vi "GUI_Preamp2_delay.vi"(8 "error IO":errorcluster) -> (0 "error IO 2":errorcluster)   [LabVIEW 2013]
uses:
  shared programs/GUI_Template/GUI_master/tcp_new_data_event.ctl
  shared programs/GUI_Template/GUI_master/tcp new data cluster.ctl
  DelayControl_For Multiple Channels.ctl
  channels_TypDef.ctl
  General/Device GUIs/GUI_DG645/DelayControl2.ctl
  VIremote/VIremote.llb/VIremoteFunction.ctl
panel:
  in  "insert tag":bool=TRUE
  in  "stop":bool
  out "status":bool
  in  "reference.Channel_D::2":string caption="reference.Channel_A::2"
  in  "reference.Channel_C::2":string caption="reference.Channel_A::2"
  in  "reference.Channel_B::2":string caption="reference.Channel_A::2"
  in  "delay.Channel_D::2":dbl=0.001 caption="Q Switch Delay" min=0.0 max=1.0 format="%_12f"
  in  "delay.Channel_C::2":dbl=0.001 caption="Q Switch Delay" min=0.0 max=1.0 format="%_12f"
  in  "Delay.Ch D":T1={"Channel"="D", "Linked"=enum."T0", "Delay"=0.0} {"Delay" format="%+.12f"}
  in  "Delay.Ch C":T1={"Channel"="C", "Linked"=enum."T0", "Delay"=0.0} {"Delay" format="%+.12f"}
  in  "Delay.Ch B":T1={"Channel"="B", "Linked"=enum."T0", "Delay"=0.0} {"Delay" format="%+.12f"}
  in  "reference.Channel_A::2":string
  in  "Delay.Ch A":T1={"Channel"="A", "Linked"=enum."T0", "Delay"=0.0} {"Delay" format="%+.12f"}
  in  "delay.Channel_A::2":dbl=0.001 caption="Lamp Delay" min=0.0 max=1.0 format="%_12f"
  in  "delay.Channel_B::2":dbl=0.001 caption="Q Switch Delay" min=0.0 max=1.0 format="%_12f"
  in  "GUIdevice 2":string="TREX-Preamp2Delay"
  out "tcp data event":T4
  # "Preamp 2"
  # "in meters..."
  # "="
  # "="
  # "="
  # "="
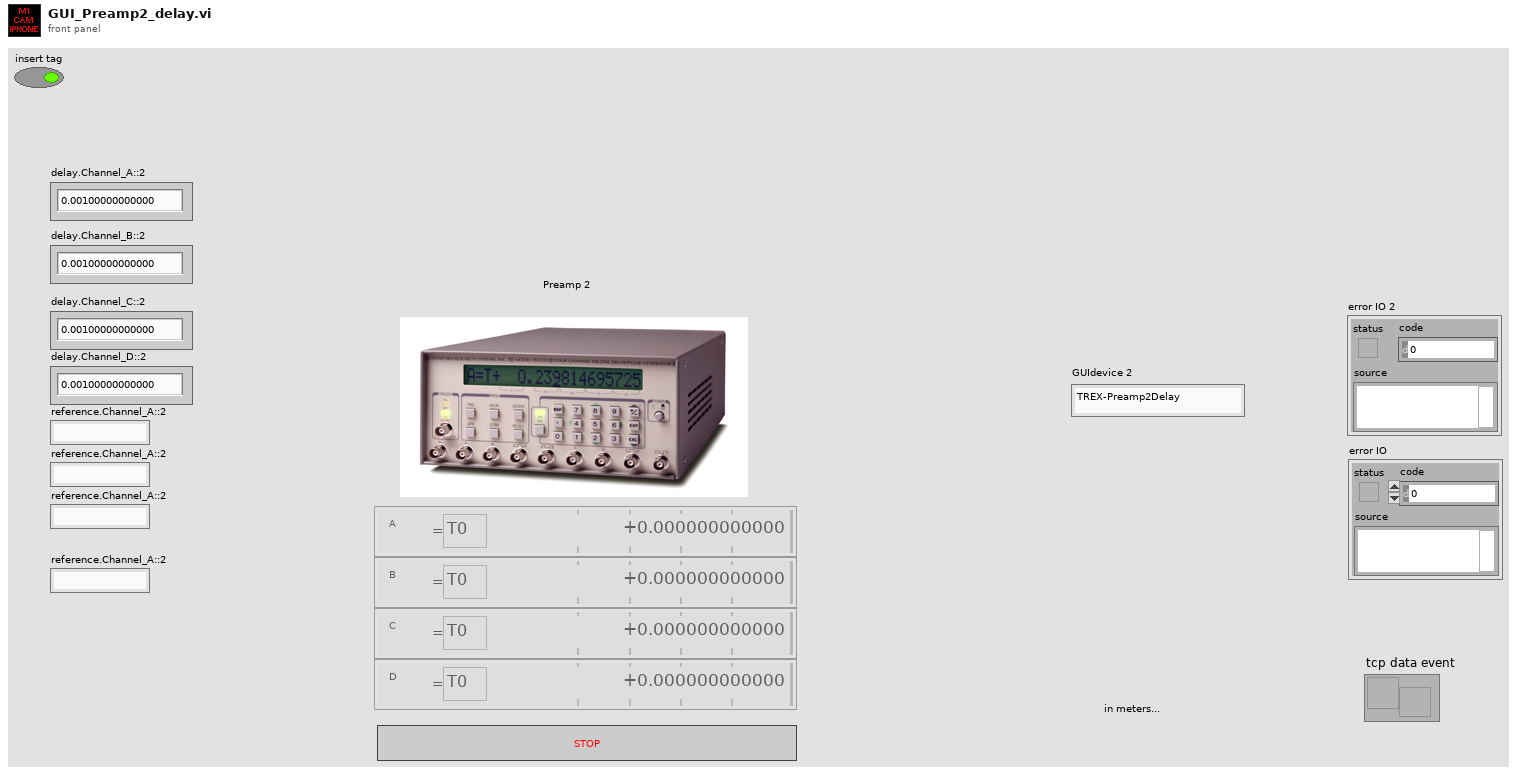
[diagram p1: front panel]
types:
  T1 = typedef "DelayControl_For Multiple Channels.ctl" = cluster{"Channel":string, "Linked":T2, "Delay":T3}
  T2 = typedef "channels_TypDef.ctl" = enum16{"T0", "A", "B", "C", "D"}
  T3 = typedef "DelayControl2.ctl" = dbl
  T4 = typedef "tcp_new_data_event.ctl" = refnum<user-event>
  T5 = typedef "tcp new data cluster.ctl" = cluster{"EventEnum":enum16{"new data", "connection status update"}, "Device name":string}
  T6 = typedef "VIremoteFunction.ctl" = enum16{"Do nothing", "Stop controller", "Close this connection", "Show info panel", "Set VI to control", "Set Accelerometer freq (Hz)", "Show Alert message", "Start Sound Input", "Stop Sound Input", "Set Volume (0-100)", "Set sound output Speaker", "Set sound output Receiver", "Play Sound", "Repeat Sound", "Stop Sound", "Pause Sound", "Resume Sound", "Set panel width of caller (320 or 480)", "Set Panel Size to Portrait", "Set Panel Size to Landscape", "Set Panel Size as Current Orientation", "Allow all UI Orientations", "Send user notification", "Disable Scrolling", "Normal Scrolling", "Page Scrolling", "Set Scroll Offset", "Page Indicator Position"}
  T7 = enum8{"Enabled", "Disabled", "Disabled and Grayed Out"}
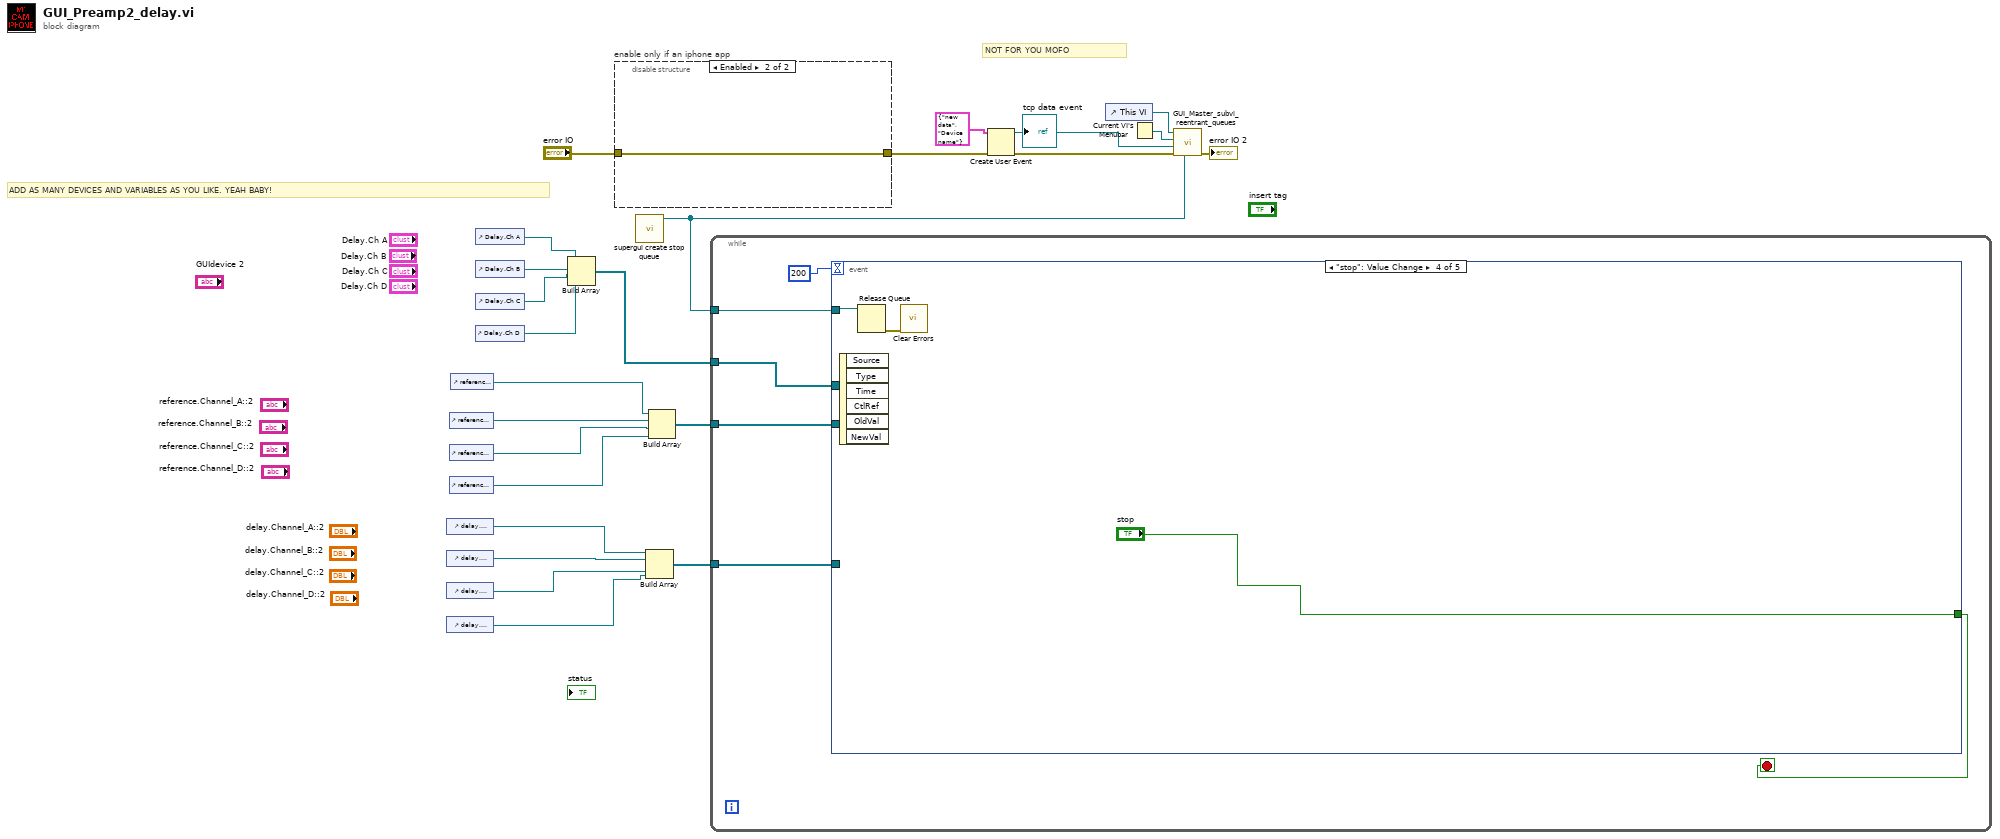
[diagram p0: block diagram]
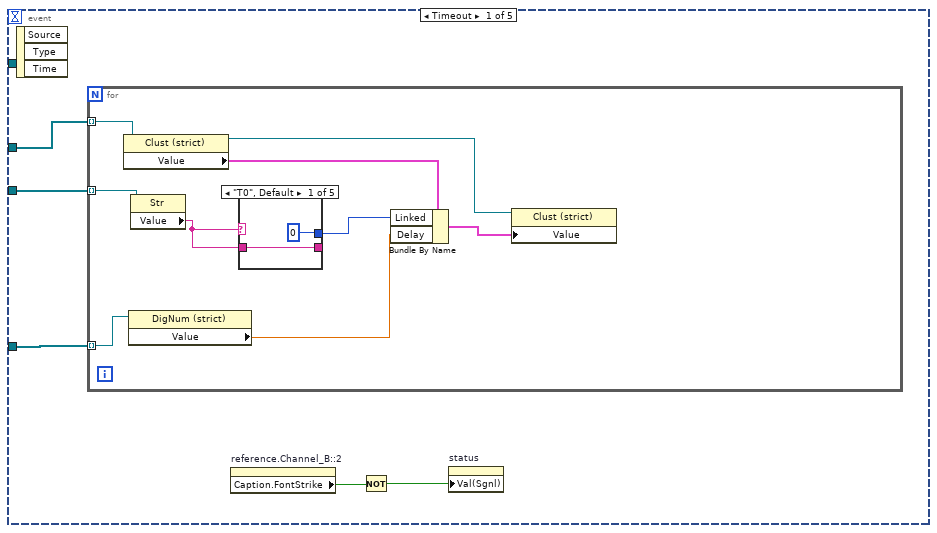
[diagram p2: hidden frame]
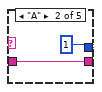
[diagram p3: hidden frame]
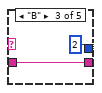
[diagram p4: hidden frame]
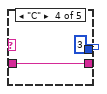
[diagram p5: hidden frame]
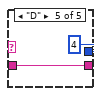
[diagram p6: hidden frame]
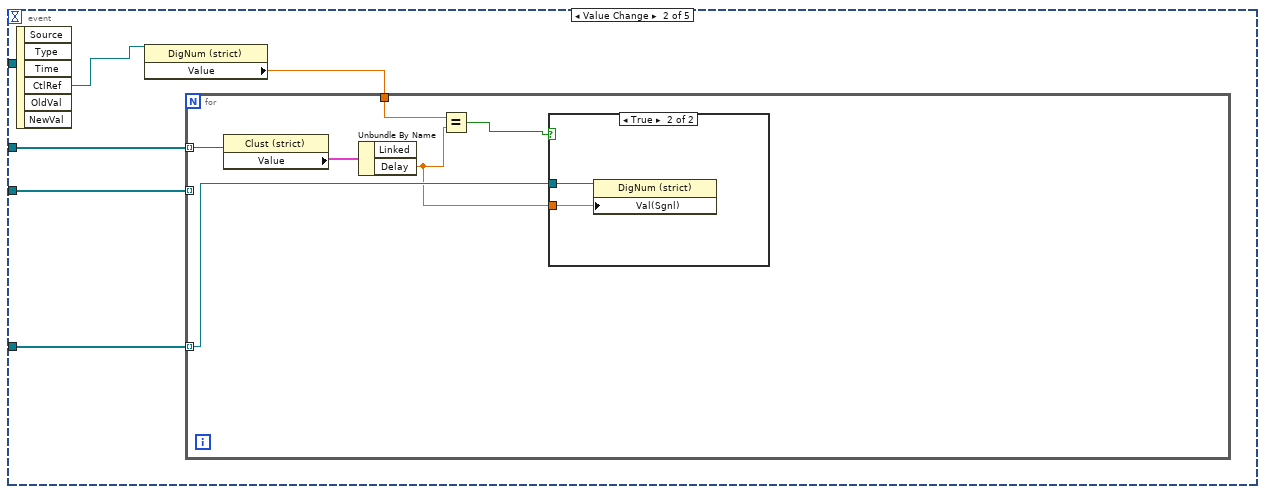
[diagram p7: hidden frame]
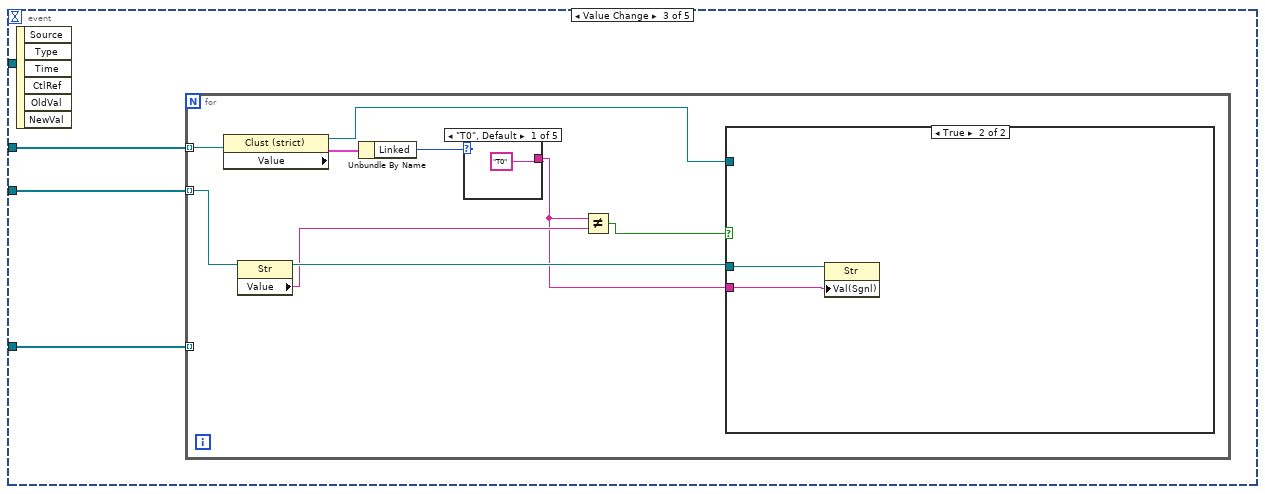
[diagram p9: hidden frame]
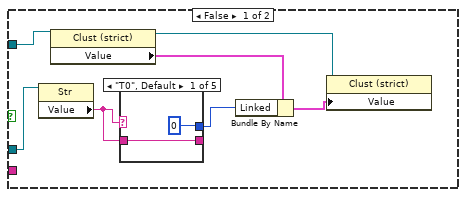
[diagram p10: hidden frame]
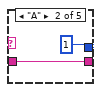
[diagram p11: hidden frame]
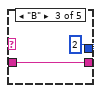
[diagram p12: hidden frame]
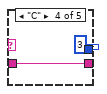
[diagram p13: hidden frame]
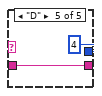
[diagram p14: hidden frame]
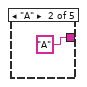
[diagram p15: hidden frame]
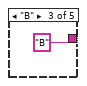
[diagram p16: hidden frame]
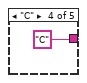
[diagram p17: hidden frame]
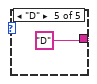
[diagram p18: hidden frame]
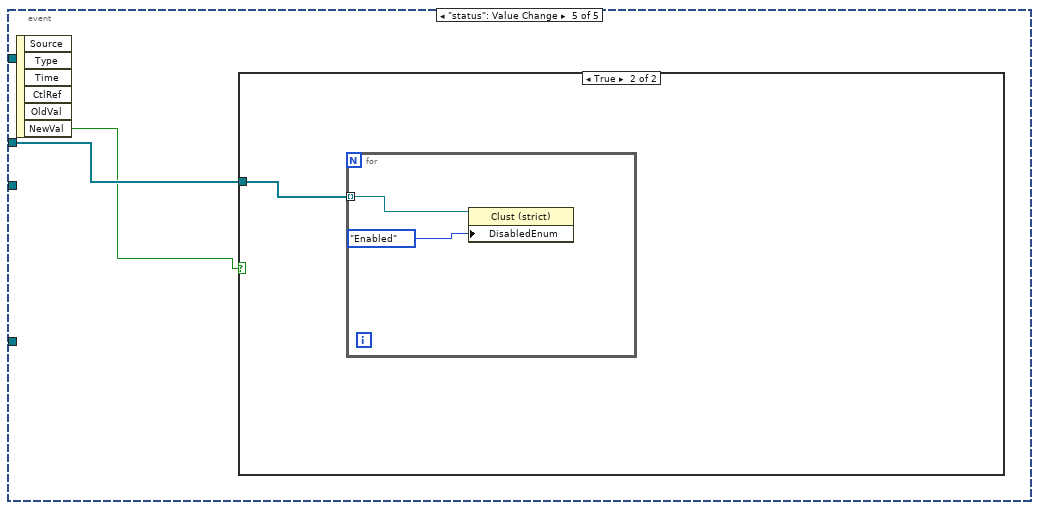
[diagram p19: hidden frame]
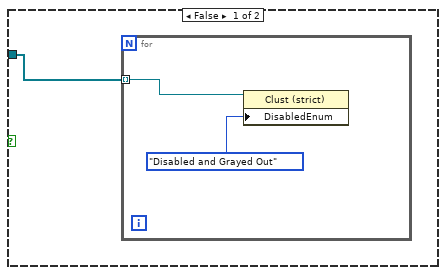
[diagram p20: hidden frame]
diagram:
  # "NOT FOR YOU MOFO"
  # "ADD AS MANY DEVICES AND VARIABLES AS YOU LIKE. YEAH BABY!"
  n1 = control-ref of="delay.Channel_A::2"() -> (w13:refnum<vi>)
  n2 = control-ref of="delay.Channel_B::2"() -> (w12:refnum<vi>)
  n3 = control-ref of="delay.Channel_C::2"() -> (w11:refnum<vi>)
  n4 = control-ref of="delay.Channel_D::2"() -> (w10:refnum<vi>)
  n5 = control-ref of="reference.Channel_B::2"() -> (w16:refnum<vi>)
  n6 = control-ref of="reference.Channel_C::2"() -> (w15:refnum<vi>)
  n7 = control-ref of="reference.Channel_D::2"() -> (w14:refnum<vi>)
  n8 = control-ref of="reference.Channel_A::2"() -> (w2:refnum<vi>)
  n9 = control-ref of="Delay.Ch A"() -> (w7:refnum<vi>)
  n10 = control-ref of="Delay.Ch B"() -> (w6:refnum<vi>)
  n11 = control-ref of="Delay.Ch C"() -> (w5:refnum<vi>)
  n12 = control-ref of="Delay.Ch D"() -> (w4:refnum<vi>)
  n13 = Build Array(w7, w6, w5, w4) -> (w3:refnum<vi>[])
  n14 = disable-structure "enable only if an iphone app" shown="Enabled" {
    disable-tunnel: [w26 w30] -> w19
    disable-tunnel: "error IO" -> [w25 w30]
    frame Disabled {
      n15 = call "VIremoteFunctions.vi"("error in (no error)"=w25, "Function"=VIremoteFunction."Set VI to control") -> ("error out"=w27:errorcluster)  [unwired: 4 in, 5 out]
      n16 = call "VIremoteFunctions.vi"("error in (no error)"=w27, "Function"=VIremoteFunction."Set Panel Size to Landscape") -> ("error out"=w26:errorcluster)  [unwired: 4 in, 5 out]
    }
    frame Enabled {
    }
  }
  n17 = call "supergui create stop queue.vi"() -> ("STOP Queue out"=w1:refnum<queue>)  [unwired: 11 in]
  n18 = Build Array(w13, w12, w11, w10) -> (w8:refnum<vi>[])
  n19 = Build Array(w2, w16, w15, w14) -> (w9:refnum<vi>[])
  n20 = while {
    tunnel: w9 -> [w34]
    tunnel: w8 -> [w33]
    tunnel: w3 -> [w32]
    tunnel: w1 -> [w31]
    stop <- w36 stop-if-true
    n21 = event shown="[3] \"stop\": Value Change" {
      selector: _ -> [_ _ _ _ _]
      dyn-events: _ -> [_ _ _ _ _]
      timeout: 200 -> [_ _ _ _ _]
      tunnel: [_ _ _ "stop" _] -> w36
      tunnel: w34 -> [w41 w64 w75 _ _]
      tunnel: w33 -> [w39 w63 w74 _ _]
      tunnel: w32 -> [w40 w65 w76 _ w114]
      tunnel: w31 -> [_ _ _ w111 _]
      event Timeout {
        n22 = event-data() -> ()  [unwired: 1 in, 3 out]
        n23 = for {
          tunnel: w41 -> [w50] mode=indexing
          tunnel: w40 -> [w49] mode=indexing
          tunnel: w39 -> [w45] mode=indexing
          n24 = property class="Clust (strict)"(reference=w49) -> (reference out=w42:refnum<vi>, "Value"=w47:T1)  [unwired: 1 in, 1 out]
          n25 = property class="DigNum (strict)"(reference=w45) -> ("Value"=w44:dbl)  [unwired: 1 in, 2 out]
          n26 = property class="Str"(reference=w50) -> ("Value"=w48:string)  [unwired: 1 in, 2 out]
          n27 = case shown="\"T0\", Default" w48 {
            tunnel: [0 1 2 3 4] -> w46
            tunnel: w48 -> [w51 w53 w55 w57 w59]
            tunnel: [w51 w53 w55 w57 w59] -> _
            frame "T0", Default {
            }
            frame "A" {
            }
            frame "B" {
            }
            frame "C" {
            }
            frame "D" {
            }
          }
          n28 = Bundle By Name(cluster=w47, "Linked"=w46, "Delay"=w44) -> (w43:T1)
          n29 = property class="Clust (strict)"(reference=w42, "Value"=w43) -> ()  [unwired: 1 in, 2 out]
        }
        n30 = property on="reference.Channel_B::2" class="Str"() -> ("Caption.FontStrike"=w38:bool)  [unwired: 2 in, 2 out]
        n31 = Not(x=w38) -> (.not. x?=w37:bool)
        n32 = property on="status" class="Bool (strict)"("Val(Sgnl)"=w37) -> ()  [unwired: 2 in, 2 out]
      }
      event Value Change {
        n33 = event-data() -> ("CtlRef"=w62:refnum<vi>)  [unwired: 1 in, 5 out]
        n34 = property class="DigNum (strict)"(reference=w62) -> ("Value"=w61:T3)  [unwired: 1 in, 2 out]
        n35 = for {
          tunnel: w65 -> [w69] mode=indexing
          tunnel: w64 -> [_] mode=indexing
          tunnel: w63 -> [w71] mode=indexing
          tunnel: w61 -> [w68]
          n36 = property class="Clust (strict)"(reference=w69) -> ("Value"=w70:T1)  [unwired: 1 in, 2 out]
          n37 = Unbundle By Name(w70) -> ("Delay"=w67:T3)  [unwired: 1 out]
          n38 = Equal?(x=w68, y=w67) -> (x = y?=w66:bool)
          n39 = case shown="True" w66 {
            tunnel: w71 -> [_ w73]
            tunnel: w67 -> [_ w72]
            frame False {
            }
            frame True {
              n40 = property class="DigNum (strict)"(reference=w73, "Val(Sgnl)"=w72) -> ()  [unwired: 1 in, 2 out]
            }
          }
        }
      }
      event Value Change {
        n41 = event-data() -> ()  [unwired: 1 in, 6 out]
        n42 = for {
          tunnel: w76 -> [w78] mode=indexing
          tunnel: w75 -> [w84] mode=indexing
          tunnel: w74 -> [_] mode=indexing
          n43 = property class="Clust (strict)"(reference=w78) -> (reference out=w77:refnum<vi>, "Value"=w79:T1)  [unwired: 1 in, 1 out]
          n44 = property class="Str"(reference=w84) -> (reference out=w83:refnum<vi>, "Value"=w82:string)  [unwired: 1 in, 1 out]
          n45 = Unbundle By Name(w79) -> ("Linked"=w85:T2)
          n46 = case shown="\"T0\", Default" w85 {
            tunnel: ["T0" "A" "B" "C" "D"] -> w80
            frame "T0", Default {
            }
            frame "A" {
            }
            frame "B" {
            }
            frame "C" {
            }
            frame "D" {
            }
          }
          n47 = Not Equal?(x=w80, y=w82) -> (x != y?=w81:bool)
          n48 = case shown="True" w81 {
            tunnel: w83 -> [w92 w104]
            tunnel: w80 -> [_ w103]
            tunnel: w77 -> [w86 _]
            frame False {
              n49 = property class="Str"(reference=w92) -> ("Value"=w90:string)  [unwired: 1 in, 2 out]
              n50 = property class="Clust (strict)"(reference=w86) -> (reference out=w88:refnum<vi>, "Value"=w91:T1)  [unwired: 1 in, 1 out]
              n51 = case shown="\"T0\", Default" w90 {
                tunnel: [0 1 2 3 4] -> w89
                tunnel: w90 -> [w93 w95 w97 w99 w101]
                tunnel: [w93 w95 w97 w99 w101] -> _
                frame "T0", Default {
                }
                frame "A" {
                }
                frame "B" {
                }
                frame "C" {
                }
                frame "D" {
                }
              }
              n52 = Bundle By Name(cluster=w91, "Linked"=w89) -> (w87:T1)
              n53 = property class="Clust (strict)"(reference=w88, "Value"=w87) -> ()  [unwired: 1 in, 2 out]
            }
            frame True {
              n54 = property class="Str"(reference=w104, "Val(Sgnl)"=w103) -> ()  [unwired: 1 in, 2 out]
            }
          }
        }
      }
      event "stop": Value Change {
        n55 = event-data() -> ()  [unwired: 1 in, 6 out]
        n56 = Release Queue(queue=w111) -> (error out=w110:errorcluster)  [unwired: 2 in, 2 out]
        n57 = call <vilib>:"Clear Errors.vi"("error in (no error)"=w110) -> ()  [unwired: 6 in, 1 out]
      }
      event "status": Value Change {
        n58 = event-data() -> ("NewVal"=w113:bool)  [unwired: 1 in, 5 out]
        n59 = case shown="True" w113 {
          tunnel: w114 -> [w115 w118]
          frame False {
            n60 = for {
              tunnel: w115 -> [w117] mode=indexing
              n61 = property class="Clust (strict)"(reference=w117, "DisabledEnum"=T7."Disabled and Grayed Out" ("Disabled")) -> ()  [unwired: 1 in, 2 out]
            }
          }
          frame True {
            n62 = for {
              tunnel: w118 -> [w120] mode=indexing
              n63 = property class="Clust (strict)"(reference=w120, "DisabledEnum"=T7."Enabled" ("Disabled")) -> ()  [unwired: 1 in, 2 out]
            }
          }
        }
      }
    }
  }
  n64 = Create User Event(user event datatype=T5 {"EventEnum"=enum."new data", "Device name"="Device name"} ("New Event"), error in=w19) -> (user event=w17:refnum<user-event>, error out=w20:errorcluster)
  "tcp data event" <- w17
  n65 = control-ref of="This VI"() -> (w23:refnum<vi>)
  n66 = Current VI's Menubar() -> (w22:refnum<k9>)
  n67 = call "GUI_Master_subvi_reentrant_queues.vi"("STOP Queue in"=w1, "error in (no error)"=w20, "tcp data event"=w17, "Caller menu reference"=w22, "Caller VI ref"=w23) -> ("error out"=→"error IO 2":errorcluster)  [unwired: 6 in]
